vi "subPZplot.vi"(10 "cursor pos":cluster{"x":dbl, "y":dbl}, 11 "PZarray":T1(array[cluster])) -> (2 "stable？":bool, 3 "PZplot":cluster{"Y":dbl[], "Y":dbl[]}[](array[cluster]))   [LabVIEW 2011]
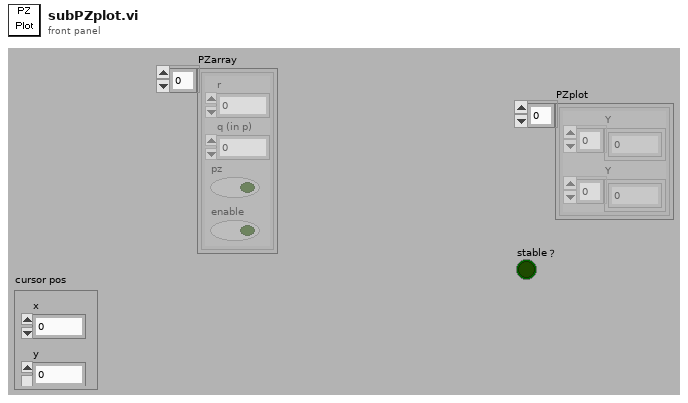
[diagram p1: front panel]
types:
  T1 = cluster{"r":dbl, "q (in p)":dbl, "pz":bool, "enable":bool}[]
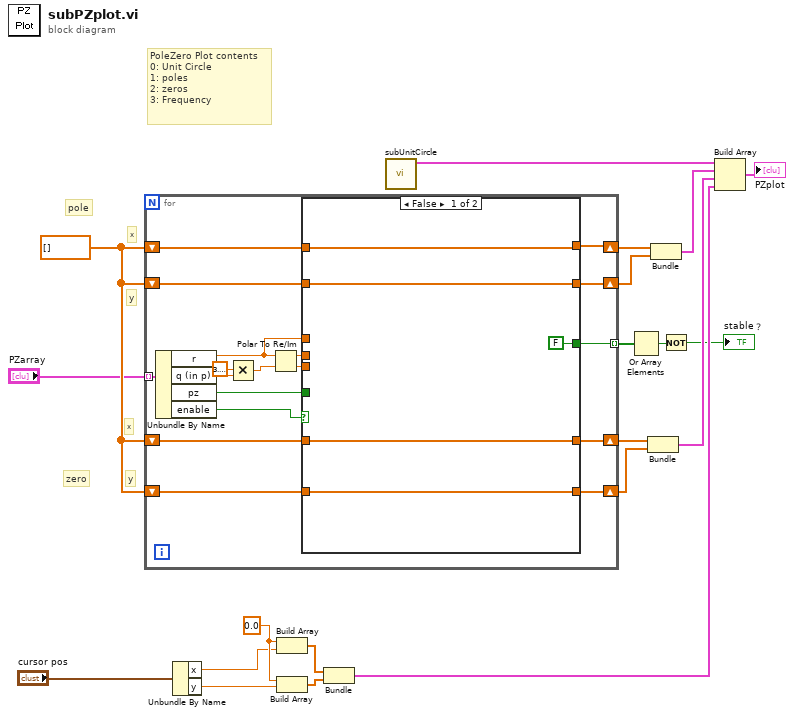
[diagram p0: block diagram]
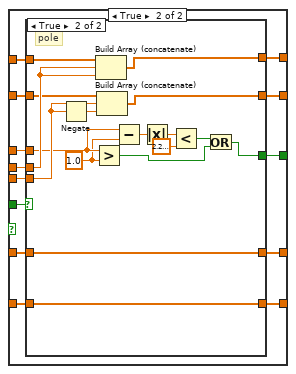
[diagram p2: hidden frame]
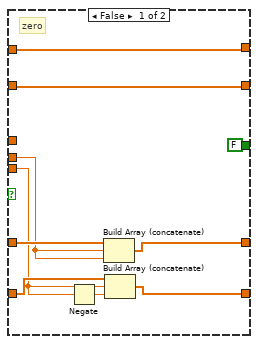
[diagram p3: hidden frame]
diagram:
  w9 = 0.0 ("element")
  w20 = dbl[] []
  # "y"
  # "x"
  # "y"
  # "x"
  # "zero"
  # "pole"
  # "PoleZero Plot contents\n0: Unit Circle\n1: poles\n2: zeros\n3: Frequency"
  n1 = for {
    tunnel: "PZarray" -> [w38] mode=indexing
    shift-right: [w30] -> w19
    shift-left: w20 -> [w31]
    shift-right: [w28] -> w18
    shift-left: w20 -> [w29]
    shift-right: [w25] -> w17
    shift-left: w20 -> [w27]
    shift-right: [w24] -> w16
    shift-left: w20 -> [w26]
    tunnel: [w22] -> w4 mode=indexing
    n2 = Unbundle By Name(w38) -> ("r"=w23:dbl, "q (in p)"=w37:dbl, "pz"=w32:bool, "enable"=w21:bool)
    n3 = Multiply(x=3.141592653589793, y=w37) -> (x*y=w35:dbl)
    n4 = Polar To Re/Im(2:w35, 3:w23) -> (0:w33:dbl, 1:w34:dbl)
    n5 = case shown="False" w21 {
      tunnel: w34 -> [_ w56]
      tunnel: w33 -> [_ w55]
      tunnel: w32 -> [_ w54]
      tunnel: w31 -> [w43 w53]
      tunnel: [w43 w52] -> w30
      tunnel: w29 -> [w42 w51]
      tunnel: [w42 w50] -> w28
      tunnel: w27 -> [w41 w49]
      tunnel: w26 -> [w40 w48]
      tunnel: [w41 w47] -> w25
      tunnel: [w40 w46] -> w24
      tunnel: w23 -> [_ w45]
      tunnel: [FALSE w44] -> w22
      frame False {
      }
      frame True {
        n6 = case shown="True" w54 {
          tunnel: w56 -> [w61 w82]
          tunnel: w55 -> [w60 w78]
          tunnel: w53 -> [w58 w83]
          tunnel: [w58 w81] -> w52
          tunnel: w51 -> [w57 w80]
          tunnel: [w57 w77] -> w50
          tunnel: w49 -> [w65 w68]
          tunnel: w48 -> [w64 w67]
          tunnel: [w63 w68] -> w47
          tunnel: [w62 w67] -> w46
          tunnel: w45 -> [_ w76]
          tunnel: [FALSE w69] -> w44
          frame False {
            # "zero"
            n7 = Negate(x=w60) -> (-x=w66:dbl)
            n8 = Build Array (concatenate)(w65, w61, w61) -> (w63:dbl[])
            n9 = Build Array (concatenate)(w64, w60, w66) -> (w62:dbl[])
          }
          frame True {
            w75 = 1.0 ("y")
            # "pole"
            n10 = Negate(x=w78) -> (-x=w79:dbl)
            n11 = Greater?(x=w76, y=w75) -> (0:w70:bool)
            n12 = Build Array (concatenate)(w83, w82, w82) -> (w81:dbl[])
            n13 = Build Array (concatenate)(w80, w78, w79) -> (w77:dbl[])
            n14 = Subtract(x=w76, y=w75) -> (x-y=w74:dbl)
            n15 = Absolute Value(x=w74) -> (abs(x)=w73:dbl)
            n16 = Less?(x=w73, y=2.220446049250313e-16) -> (x < y?=w71:bool)
            n17 = Or(x=w71, y=w70) -> (x .or. y?=w69:bool)
          }
        }
      }
    }
  }
  n18 = Unbundle By Name("cursor pos") -> ("x"=w7:dbl, "y"=w8:dbl)
  n19 = Build Array(w9, w7) -> (w10:dbl[])
  n20 = Build Array(w9, w8) -> (w11:dbl[])
  n21 = Bundle(w10, w11) -> (w5:cluster{dbl[], dbl[]})  [unwired: 1 in]
  n22 = call "subUnitCircle.vi"() -> ("XY Graph"=w15:cluster{"Y":dbl[], "Y":dbl[]})  [unwired: 11 in]
  n23 = Or Array Elements(Boolean array=w4) -> (logical OR=w3:bool)
  n24 = Bundle(w17, w16) -> (w13:cluster{dbl[], dbl[]})  [unwired: 1 in]
  n25 = Bundle(w19, w18) -> (w14:cluster{dbl[], dbl[]})  [unwired: 1 in]
  n26 = Not(x=w3) -> (.not. x?=→"stable？":bool)
  n27 = Build Array(w15, w14, w13, w5) -> (→"PZplot":cluster{"Y":dbl[], "Y":dbl[]}[])
